vi "obliczOdleglosc.vi"(7 "Promień [m]":dbl, 8 "P2":i32[](array[numeric]), 11 "P1":i32[](array[numeric])) -> (3 "Odległość [m]":dbl format="%_4g")   [LabVIEW 2014]
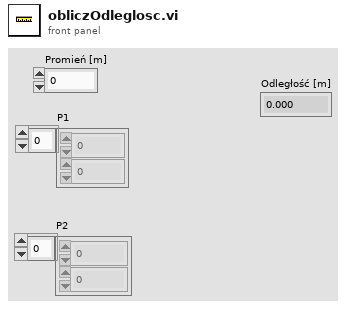
[diagram p1: front panel]
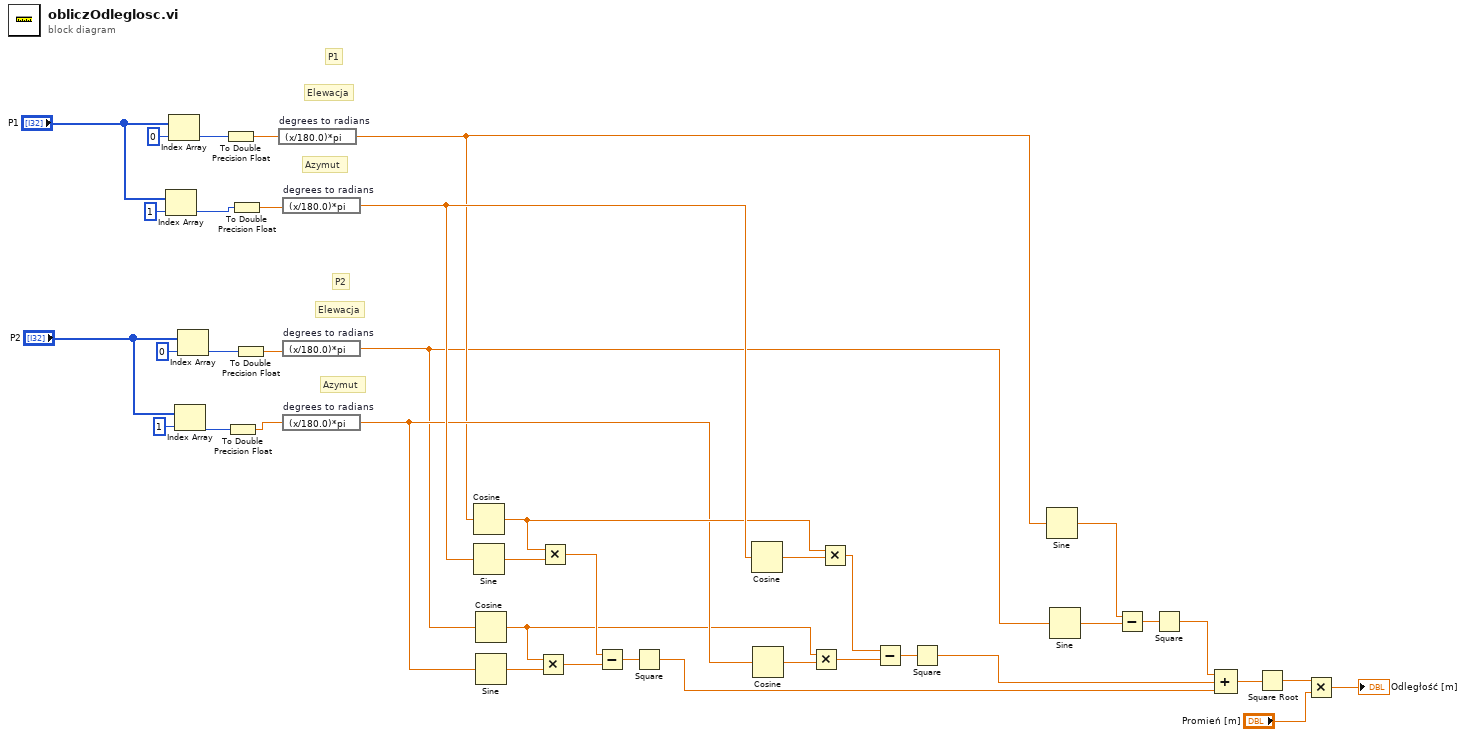
[diagram p0: block diagram]
diagram:
  # "P2"
  # "P1"
  # "Azymut"
  # "Elewacja"
  # "Azymut"
  # "Elewacja"
  n1 = Index Array(array="P1", index=1) -> (element=w27:i32)
  n2 = Index Array(array="P1", index=0) -> (element=w34:i32)
  n3 = Index Array(array="P2", index=1) -> (element=w28:i32)
  n4 = Index Array(array="P2", index=0) -> (element=w29:i32)
  n5 = To Double Precision Float(number=w34) -> (double precision float=w33:dbl)
  n6 = To Double Precision Float(number=w28) -> (double precision float=w30:dbl)
  n7 = To Double Precision Float(number=w27) -> (double precision float=w32:dbl)
  n8 = To Double Precision Float(number=w29) -> (double precision float=w31:dbl)
  n9 = expression code="(x/180.0)*pi" "degrees to radians"(w33) -> (w12:dbl)
  n10 = expression code="(x/180.0)*pi" "degrees to radians"(w32) -> (w21:dbl)
  n11 = expression code="(x/180.0)*pi" "degrees to radians"(w31) -> (w11:dbl)
  n12 = expression code="(x/180.0)*pi" "degrees to radians"(w30) -> (w18:dbl)
  n13 = Cosine(x=w12) -> (cos(x)=w19:dbl)
  n14 = Sine(x=w21) -> (sin(x)=w26:dbl)
  n15 = Cosine(x=w11) -> (cos(x)=w16:dbl)
  n16 = Sine(x=w18) -> (sin(x)=w25:dbl)
  n17 = Multiply(x=w16, y=w25) -> (x*y=w23:dbl)
  n18 = Multiply(x=w19, y=w26) -> (x*y=w24:dbl)
  n19 = Subtract(x=w24, y=w23) -> (x-y=w22:dbl)
  n20 = Square(x=w22) -> (x^2=w5:dbl)
  n21 = Cosine(x=w21) -> (cos(x)=w20:dbl)
  n22 = Cosine(x=w18) -> (cos(x)=w17:dbl)
  n23 = Multiply(x=w16, y=w17) -> (x*y=w14:dbl)
  n24 = Multiply(x=w19, y=w20) -> (x*y=w13:dbl)
  n25 = Subtract(x=w13, y=w14) -> (x-y=w15:dbl)
  n26 = Square(x=w15) -> (x^2=w6:dbl)
  n27 = Sine(x=w12) -> (sin(x)=w8:dbl)
  n28 = Sine(x=w11) -> (sin(x)=w9:dbl)
  n29 = Subtract(x=w8, y=w9) -> (x-y=w10:dbl)
  n30 = Square(x=w10) -> (x^2=w7:dbl)
  n31 = Compound Arithmetic op=ADD(w7, w6, w5) -> (w4:dbl)
  n32 = Square Root(x=w4) -> (sqrt(x)=w3:dbl)
  n33 = Multiply(x=w3, y="Promień [m]") -> (x*y=→"Odległość [m]":dbl)
